vi "girpcutil_connect_disconnect.vi"(6 "timeout":u32, 7 "Connect":bool=TRUE, 8 "Fehler (Eingang, kein Fehler)":errorcluster, 9 "port":u32=8090, 10 "host":string="127.0.0.1", 11 "girpcutil_params":T1={"ConnectionHandle"=-1, "DLL-Handle"={"DLL Path"=path "C:/Users/wernerj-test/Desktop/labview xmlrpc/DLL/DLL/64bit/girpcutil.dll", "Is32Bit"=FALSE}}) -> (0 "Fehler (Ausgang)":errorcluster, 3 "girpcutil_params 2":T1)   [LabVIEW 2016]
uses:
  girpcutil_params.ctl
panel:
  out "Rückgabewert":i32
  out "Rückgabewert 2":i32
  out "errMsgLen":i32
  out "errMsg":u8[](array[numeric])
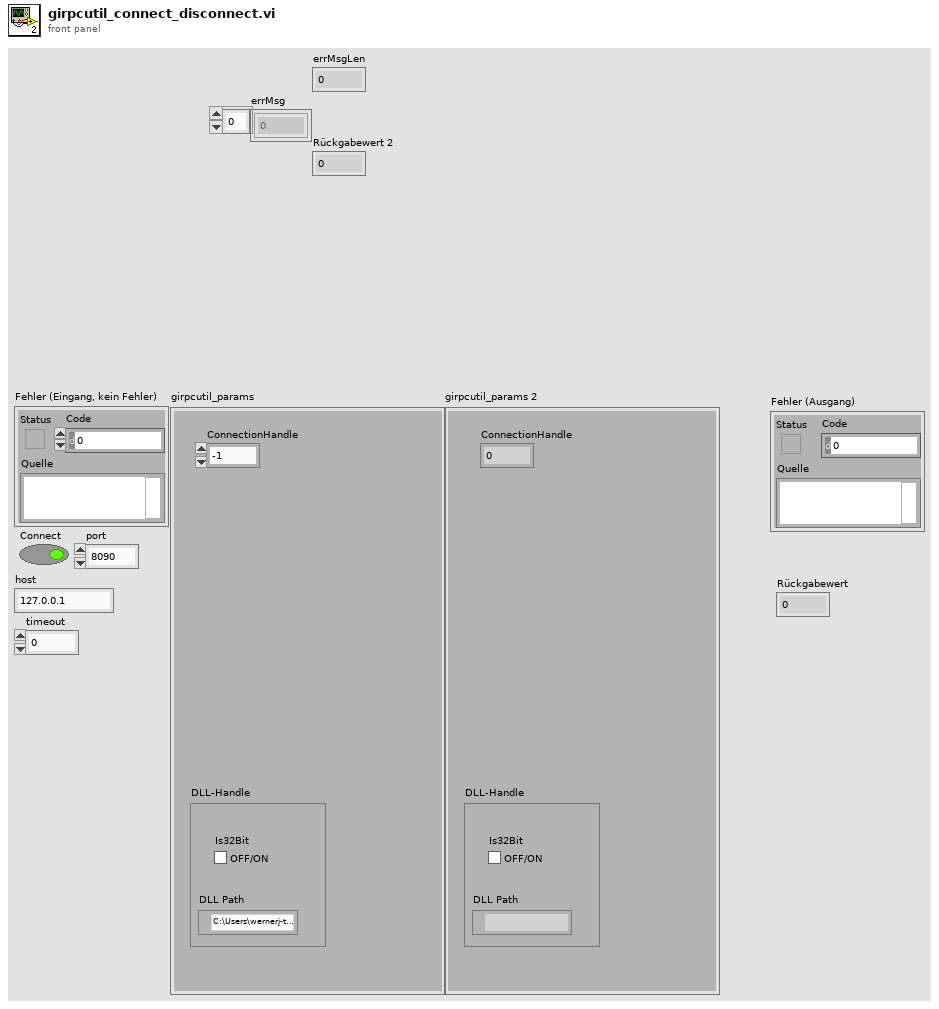
[diagram p1: front panel]
types:
  T1 = typedef "girpcutil_params.ctl" = cluster{"ConnectionHandle":i32, "DLL-Handle":cluster{"DLL Path":path, "Is32Bit":bool}}
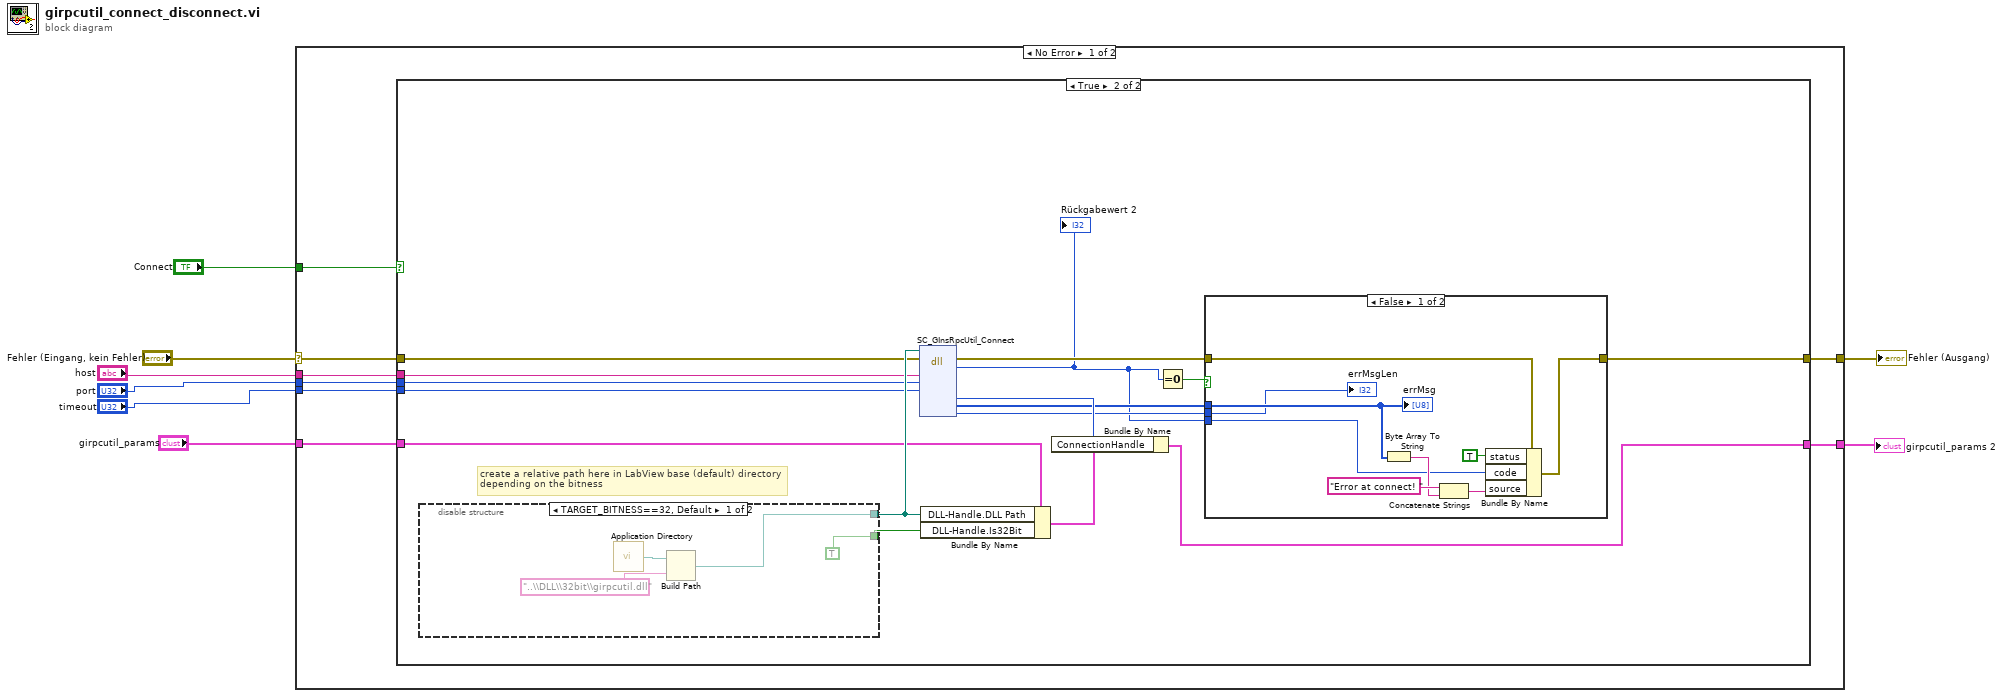
[diagram p0: block diagram]
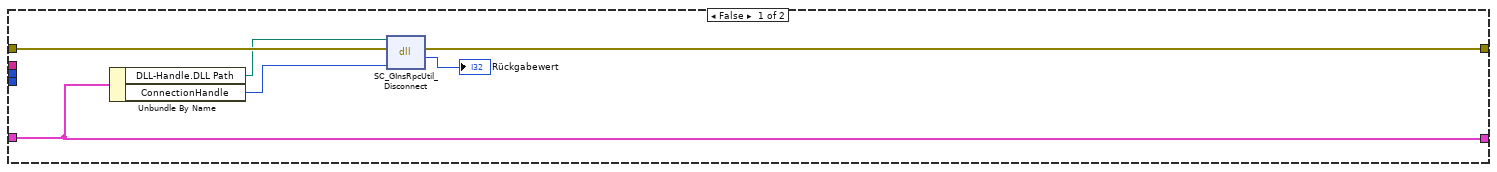
[diagram p2: hidden frame]
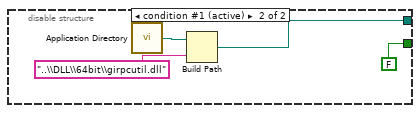
[diagram p4: hidden frame]
diagram:
  n1 = case shown="No Error" "Fehler (Eingang, kein Fehler)" {
    selector: "Fehler (Eingang, kein Fehler)" -> [w15 w57]
    tunnel: [w13 w57] -> w7
    tunnel: "girpcutil_params" -> [w14 _]
    tunnel: "Connect" -> [w16 _]
    tunnel: [w12 _] -> w4
    tunnel: "host" -> [w11 _]
    tunnel: "timeout" -> [w10 _]
    tunnel: "port" -> [w9 _]
    frame No Error {
      n2 = case shown="True" w16 {
        tunnel: w15 -> [w21 w35]
        tunnel: w14 -> [w17 w34]
        tunnel: [w18 w27] -> w13
        tunnel: [w17 w26] -> w12
        tunnel: w11 -> [_ w32]
        tunnel: w10 -> [_ w31]
        tunnel: w9 -> [_ w30]
        frame False {
          n3 = Unbundle By Name(w17) -> ("DLL-Handle.DLL Path"=w19:path, "ConnectionHandle"=w20:i32)
          n4 = dll-call lib="?" fn="SC_GInsRpcUtil_Disconnect"(path in=w19, error in=w21, "connectionHandle"=w20) -> (error out=w18:errorcluster, "Rückgabewert"=→"Rückgabewert":i32)  [unwired: 2 in, 1 out]
        }
        frame True {
          # "create a relative path here in LabView base (default) directory\ndepending on the bitness"
          n5 = disable-structure shown="TARGET_BITNESS==32, Default" {
            disable-tunnel: [w49 w53] -> w37
            disable-tunnel: [TRUE ("DLL-Handle.Is32Bit") FALSE ("DLL-Handle.Is32Bit")] -> w38
            frame condition #0 {
              n6 = call <vilib>:"Application Directory.vi"() -> ("Application Directory"=w51:path)
              n7 = Build Path(base path=w51, name or relative path="..\\DLL\\32bit\\girpcutil.dll") -> (appended path=w49:path)
            }
            frame condition #1 (active) {
              n8 = call <vilib>:"Application Directory.vi"() -> ("Application Directory"=w55:path)
              n9 = Build Path(base path=w55, name or relative path="..\\DLL\\64bit\\girpcutil.dll") -> (appended path=w53:path)
            }
          }
          n10 = dll-call lib="?" fn="SC_GInsRpcUtil_Connect"(path in=w37, error in=w35, "host"=w32, "port"=w30, "timeout"=w31) -> (error out=w28:errorcluster, "Rückgabewert"=w23:i32, "connectionHandle"=w36:i32, "errMsg"=w25:u8[], "errMsgLen"=w24:i32)  [unwired: 7 in, 1 out]
          "Rückgabewert 2" <- w23
          n11 = Bundle By Name(cluster=w34, "DLL-Handle.DLL Path"=w37, "DLL-Handle.Is32Bit"=w38) -> (w33:T1)
          n12 = Bundle By Name(cluster=w33, "ConnectionHandle"=w36) -> (w26:T1)
          n13 = Equal To 0?(x=w23) -> (x = 0?=w29:bool)
          n14 = case shown="False" w29 {
            tunnel: w28 -> [w41 w48]
            tunnel: [w40 w48] -> w27
            tunnel: w25 -> [w45 _]
            tunnel: w24 -> [w42 _]
            tunnel: w23 -> [w39 _]
            frame False {
              n15 = Byte Array To String(unsigned byte array=w45) -> (string=w46:string)
              n16 = Concatenate Strings("Error at connect! " ("source"), w46) -> (w44:string)
              n17 = Bundle By Name(cluster=w41, "status"=TRUE, "code"=w39, "source"=w44) -> (w40:errorcluster)
              "errMsg" <- w45
              "errMsgLen" <- w42
            }
            frame True {
            }
          }
        }
      }
    }
    frame Error {
    }
  }
  "Fehler (Ausgang)" <- w7
  "girpcutil_params 2" <- w4
